vi "Get Computer Metadata.vi"(8 "error in (no error)":errorcluster) -> (0 "error out":errorcluster, 3 "Computer Metadata":T1)   [LabVIEW 2020]
doc: "This VI opens a reference to the localhost resource, gets computer OS and hardware metadata, then builds the \"Computer Metadata\" cluster from it."
uses:
  Type Definitions/Computer Metadata.ctl
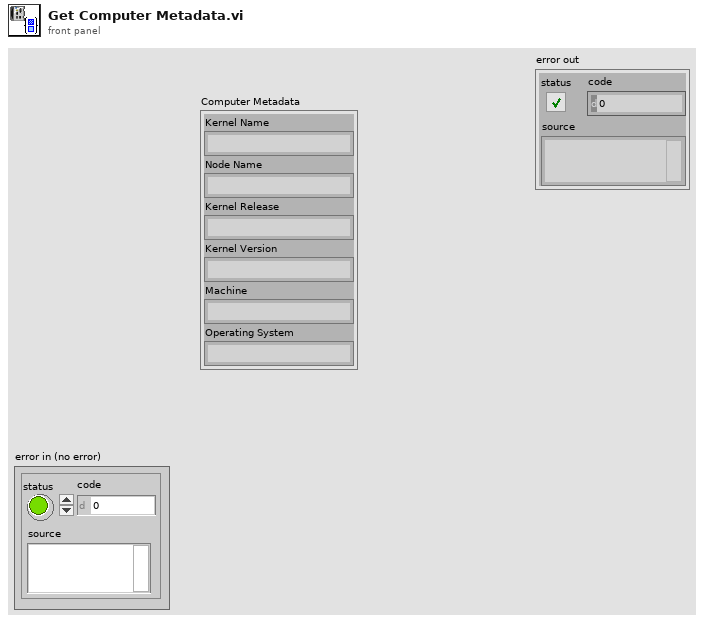
[diagram p1: front panel]
types:
  T1 = typedef "Computer Metadata.ctl" = cluster{"Kernel Name":string, "Node Name":string, "Kernel Release":string, "Kernel Version":string, "Machine":string, "Operating System":string}
  T2 = cluster{"[0]":string, "[1]":string, "[2]":string, "[3]":string, "[4]":string, "[5]":string}
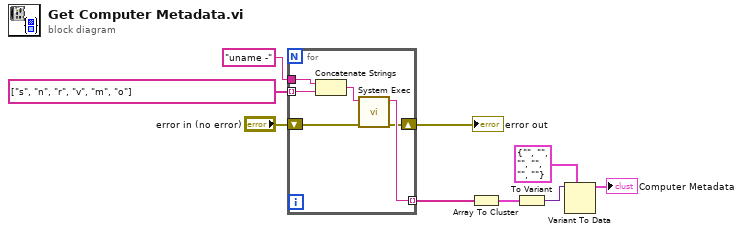
[diagram p0: block diagram]
diagram:
  n1 = for {
    tunnel: "uname -" ("command line") -> [w15]
    tunnel: [w13] -> w5 mode=indexing
    tunnel: string[] ["s", "n", "r", "v", "m", "o"] ("string") -> [w12] mode=indexing
    shift-right: [w10] -> w6
    shift-left: "error in (no error)" -> [w11]
    n2 = Concatenate Strings(w15, w12) -> (w14:string)
    n3 = call <vilib>:"System Exec.vi"("error in (no error)"=w11, "command line"=w14) -> ("error out"=w10:errorcluster, "standard output"=w13:string)  [unwired: 6 in, 2 out]
  }
  "error out" <- w6
  n4 = Array To Cluster(array=w5) -> (cluster=w4:T2)
  n5 = To Variant(anything=w4) -> (Variant=w3:variant)
  n6 = Variant To Data(type=T1 {"Kernel Name"="", "Node Name"="", "Kernel Release"="", "Kernel Version"="", "Machine"="", "Operating System"=""} ("Computer Metadata"), Variant=w3) -> (data=→"Computer Metadata":T1)  [unwired: 1 in, 1 out]
